vi "Picture Factory.vi"() -> ()   [LabVIEW 2014, in "PH_StatusHandler.lvlib"]
uses:
  PH_StatusHandler.lvlib
  PH_Common/PH_Common.lvlib
panel:
  out "picture":picture
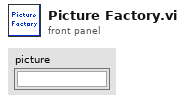
[diagram p1: front panel]
types:
  T1 = enum16{"User-specified Font", "Application Font", "System Font", "Dialog Font"}
  T2 = cluster{"Font Name:":string, "Size":i16, "Strikeout?":bool, "Italic?":bool, "Underline?":bool, "Outline?":bool, "Shadow?":bool, "Bold?":bool}
  T3 = cluster{"horizontal":enum16{"left", "center", "right"}, "vertical":enum16{"top", "center", "bottom"}}
  T4 = cluster{"left":i16, "top":i16, "right":i16, "bottom":i16}
  T5 = typedef "imagedata.ctl" = cluster{"image type":i32, "image depth":i32, "image":u8[], "mask":u8[], "colors":u32[], "Rectangle":cluster{"left":i16, "top":i16, "right":i16, "bottom":i16}}
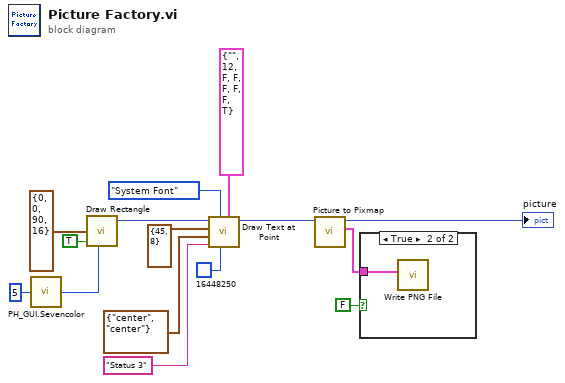
[diagram p0: block diagram]
diagram:
  n1 = call "PH_GUI.Sevencolor.vi"("State"=5) -> ("Color Box"=w11:u32)
  n2 = call <vilib>:"Draw Rectangle.vi"("rect"=T4 {"left"=0, "top"=0, "right"=90, "bottom"=16}, "fill?(F)"=TRUE, "color(black)"=w11) -> ("new picture"=w13:picture)  [unwired: 6 in]
  n3 = call <vilib>:"Draw Text at Point.vi"("[user-specified font]"=T2 {"Font Name:"="", "Size"=12, "Strikeout?"=FALSE, "Italic?"=FALSE, "Underline?"=FALSE, "Outline?"=FALSE, "Shadow?"=FALSE, "Bold?"=TRUE}, "text color(black)"=u32 16448250 ("Color Box"), "desired font(Application)"=T1."System Font", "text"="Status 3", "alignment(left, top)"=T3 {"horizontal"=enum."center", "vertical"=enum."center"}, "origin"=cluster{"x":i16, "y":i16} {"x"=45, "y"=8}, "picture"=w13) -> ("new picture"=w5:picture)  [unwired: 3 in, 1 out]
  n4 = call <vilib>:"Picture to Pixmap.vi"("picture"=w5) -> ("image data"=w3:T5, "new picture"=→"picture":picture)  [unwired: 9 in]
  n5 = case shown="True" FALSE {
    tunnel: w3 -> [_ w16]
    frame False {
    }
    frame True {
      n6 = call <vilib>:"Write PNG File.vi"("image data"=w16) -> ()  [unwired: 9 in, 2 out]
    }
  }
